vi "PRACTICA 2 CONVERSION DE UNIDADES DE TEMPERATURA.vi"() -> ()   [LabVIEW 2017]
panel:
  out "ºF":dbl
  in  "ºC":dbl
  out "ºC":dbl
  in  "ºF":dbl
  # "PRACTICA 2 CONVERSION DE UNIDADES DE TEMPERATURA"
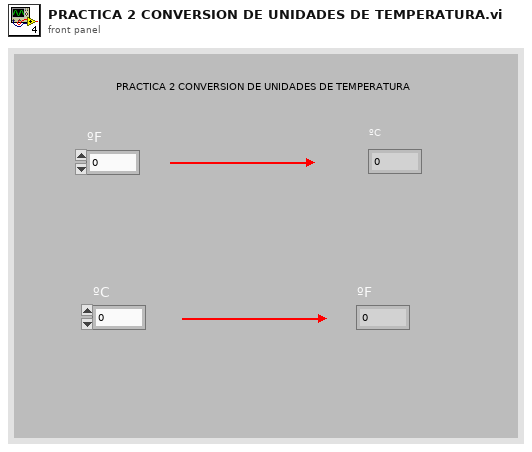
[diagram p1: front panel]
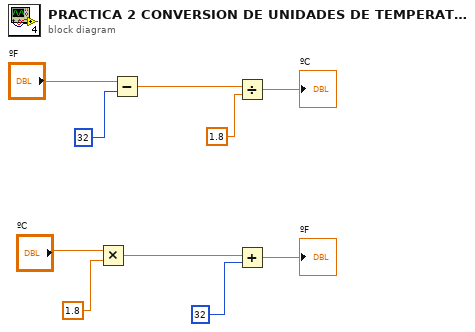
[diagram p0: block diagram]
diagram:
  n1 = Multiply(x="ºC", y=1.8) -> (x*y=w3:dbl)
  n2 = Subtract(x="ºF", y=32) -> (x-y=w7:dbl)
  n3 = Divide(x=w7, y=1.8) -> (x/y=→"ºC":dbl)
  n4 = Add(x=w3, y=32) -> (x+y=→"ºF":dbl)
